vi "post_pelletron.vi"(8 "error in (no error)":errorcluster, 11 "Pelletron Data":T1={"ID"=8, "Integer Timestamp"=2, "High Voltage"=3.0, "+ High Voltage Supply"=4.0, "- High Voltage Supply"=5.0, "HV Control Difference"=6.0, "Vacuum Pressure"=7.0, "Radiation"=8.0, "Column Current"=9.0, "Lost Charge"=54.0, "Chain Current"=3.0, "Control High Voltage"=0.0}) -> (0 "error out":errorcluster, 3 "Test Server":bool)   [LabVIEW 2013]
doc: "Adds a the given cluster to the pelletron_data table."
uses:
  Controls/Pelletron.ctl
  <vilib>/addons/database/NI_Database_API.lvlib
panel:
  # "Pelletron"
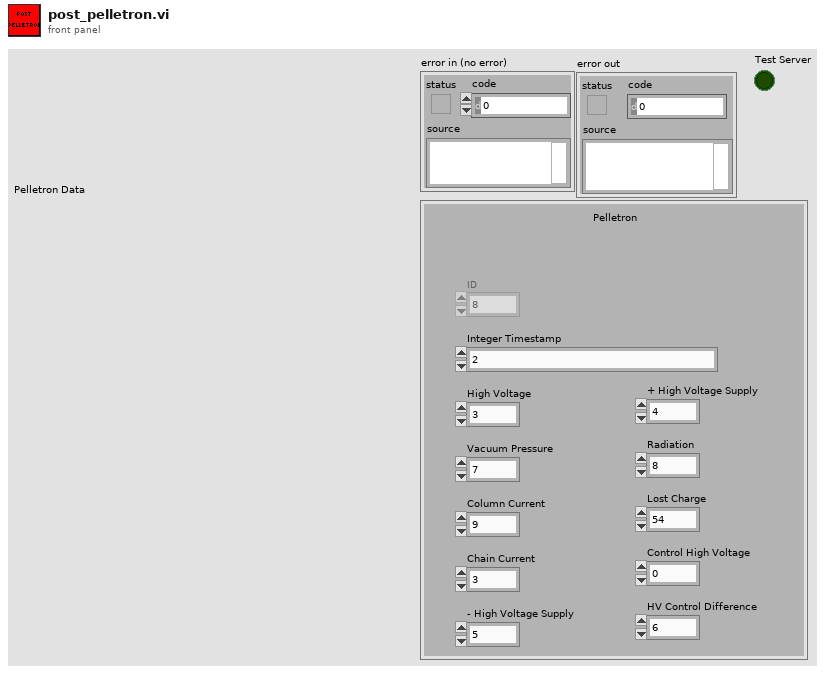
[diagram p1: front panel]
types:
  T1 = typedef "Pelletron.ctl" = cluster{"ID":i32, "Integer Timestamp":u64, "High Voltage":sgl, "+ High Voltage Supply":sgl, "- High Voltage Supply":sgl, "HV Control Difference":sgl, "Vacuum Pressure":sgl, "Radiation":sgl, "Column Current":sgl, "Lost Charge":sgl, "Chain Current":sgl, "Control High Voltage":sgl}
  T2 = typedef "NI_Database_API.lvlib/Conn ObjectReference.ctl" = refnum<k1>
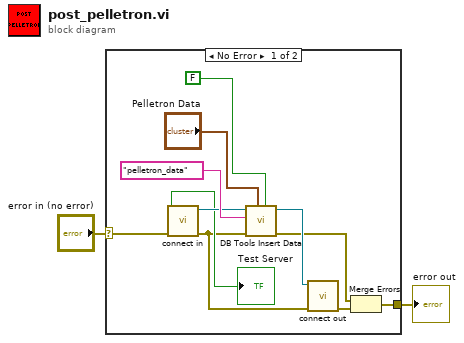
[diagram p0: block diagram]
diagram:
  n1 = case shown="No Error" "error in (no error)" {
    selector: "error in (no error)" -> [w13 w14]
    tunnel: [w3 w14] -> w1
    frame No Error {
      n2 = call "connect in.vi"("error in (no error)"=w13) -> ("error out"=w5:errorcluster, "Database Connection"=w11:T2, "Test Server"=→"Test Server":bool)  [unwired: 6 in]
      n3 = call <vilib>:"DB Tools Insert Data.vi"("create table? (F)"=FALSE, "data"="Pelletron Data", "error in (no error)"=w5, "table"="pelletron_data", "connection reference"=w11) -> ("error out"=w6:errorcluster, "connection reference out"=w10:T2)  [unwired: 5 in]
      n4 = call "connect out.vi"("error in (no error)"=w5, "connection reference"=w10) -> ("error out"=w4:errorcluster)  [unwired: 9 in]
      n5 = Merge Errors(w6, w4) -> (w3:errorcluster)
    }
    frame Error {
    }
  }
  "error out" <- w1
